vi "BooleanAlternator.vi"(9 "Initializer":bool, 10 "Boolean in":bool) -> (2 "Boolean out":bool)   [LabVIEW 2012]
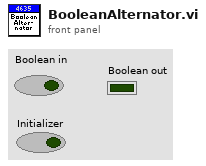
[diagram p1: front panel]
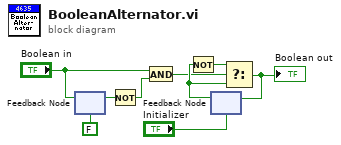
[diagram p0: block diagram]
diagram:
  n1 = feedback #1(FALSE) -> (w6:bool)
  n2 = feedback-in #1("Boolean in") -> ()
  n3 = Not(x=w6) -> (.not. x?=w5:bool)
  n4 = And(x="Boolean in", y=w5) -> (x .and. y?=w7:bool)
  n5 = feedback #2("Initializer") -> (w8:bool)
  n6 = Not(x=w8) -> (.not. x?=w9:bool)
  n7 = Select(t=w9, s=w7, f=w8) -> (s? t:f=w3:bool)
  "Boolean out" <- w3
  n8 = feedback-in #2(w3) -> ()
